vi "tdms存储.vi"() -> ()   [LabVIEW 2018]
panel:
  out "波形图表":cluster{dbl, dbl}(graph)
  in  "停止":bool
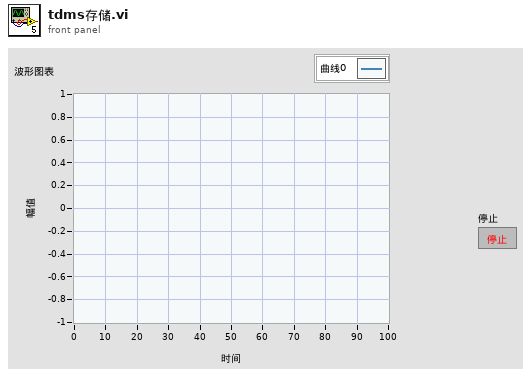
[diagram p1: front panel]
types:
  T1 = enum16{"open", "open or create", "create or replace", "create", "open (read-only)"}
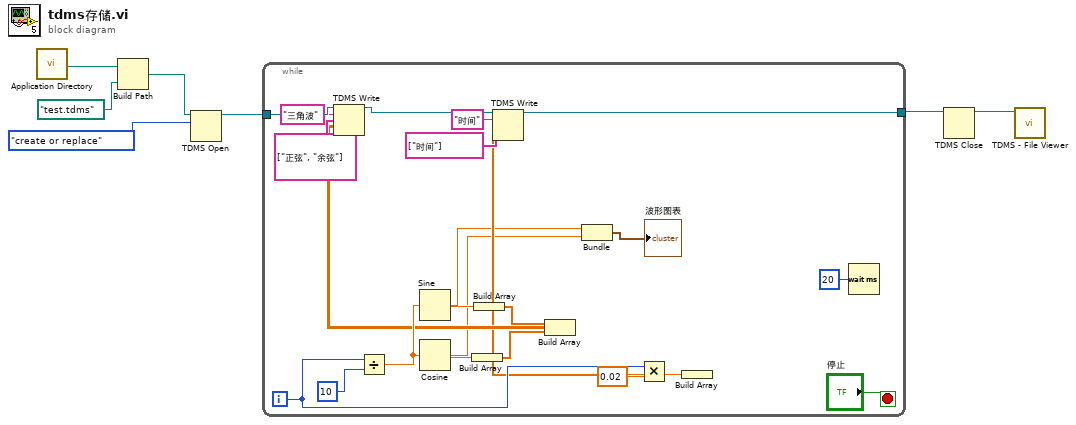
[diagram p0: block diagram]
diagram:
  n1 = call <vilib>:"Application Directory.vi"() -> ("Application Directory"=w6:path)
  n2 = Build Path(base path=w6, name or relative path=path "test.tdms") -> (appended path=w5:path)
  n3 = TDMS Open(10:T1."create or replace" ("操作(0:open)"), 11:w5) -> (3:w3:refnum<k34>)  [unwired: 5 in, 1 out]
  n4 = while {
    tunnel: w3 -> [w27]
    tunnel: [w11] -> w2
    i -> [w18]
    stop <- "停止" stop-if-true
    n5 = Divide(x=w18, y=10) -> (x/y=w23:dbl)
    n6 = Sine(x=w23) -> (sin(x)=w10:dbl)
    n7 = Cosine(x=w23) -> (cos(x)=w9:dbl)
    n8 = Build Array(w9) -> (w21:dbl[])
    n9 = Build Array(w10) -> (w22:dbl[])
    n10 = Build Array(w22, w21) -> (w20:dbl[][])
    n11 = TDMS Write(0:w27, 5:"三角波" ("组名称输入（无标题）"), 7:string[] ["正弦", "余弦"] ("通道名输入（无标题）"), 9:w20) -> (4:w16:refnum<k34>)  [unwired: 2 in, 3 out]
    n12 = Bundle(w10, w9) -> (→"波形图表":cluster{dbl, dbl})  [unwired: 1 in]
    n13 = Multiply(x=w18, y=0.02) -> (x*y=w13:dbl)
    n14 = Build Array(w13) -> (w12:dbl[])
    n15 = TDMS Write(0:w16, 5:"时间" ("组名称输入（无标题）"), 7:string[] ["时间"] ("通道名输入（无标题）"), 9:w12) -> (4:w11:refnum<k34>)  [unwired: 2 in, 3 out]
    n16 = Wait (ms)(milliseconds to wait=u32 20 ("等待时间（毫秒）")) -> ()  [unwired: 1 out]
  }
  n17 = TDMS Close(11:w2) -> (3:w1:path)  [unwired: 1 in, 1 out]
  n18 = call <vilib>:"TDMS - File Viewer.vi"("file path"=w1) -> ()  [unwired: 5 in, 2 out]
